vi "Pop-up password request.vi"(4 "error in (no error)":errorcluster, 7 "Filepath":path=path "C:/Projects - VSS/PART11 & DI TOOLKIT/passwords.log") -> (0 "error out":errorcluster, 1 "Activity log":T5 {"Epoch sec" format="%.2e"}, 2 "User access cluster":T3 {"Expire sec" format="%.2f"}, 3 "Valid password?":bool)   [LabVIEW 2013]
doc: "This is a pop-up panel which forces the user to enter a valid password or click cancel. It is a modal GUI.\n\nIt uses a filepath to an encrypted password file. If the user fails to enter a valid set of user ID and password within a set number of attempts (from the password file) the vi returns with valid password = F. \n\nIf there is a file read error then \"valid password?\" = F and a custom error code is returned (error not announced here). Conversely, incorrect user ID or password entries and expired passwords ARE announced in this vi.\n\nIt returns the User ID result, Security level (0 - 10), and an activty log of all failed and succesfull log-in attempts, which can be written to an activity log file by subsequent vis."
uses:
  User Access Type defs/Acitivity cluster array.ctl
  User Access Type defs/Acitivity cluster.ctl
  User Access Type defs/User access cluster.ctl
  User Access Type defs/Security level U8.ctl
  User Access Type defs/All users access configuration cluster.ctl
  User Access Type defs/User access cluster array.ctl
  <vilib>/Utility/miscctls.llb/LVPointTypeDef.ctl
panel:
  out "Access Configuration":T1 {"User array"."Expire sec" format="%.2f"}
  out "Lock user?":bool
  out "index":i32
  out "Password count":u8
  out "User ID count":u8
  out "State case":string
  in  "Password":string
  in  "Boolean 2":bool
  in  "Boolean":bool
  out "prompt":string="Enter a valid operator ID\nand password"
  in  "User ID":string
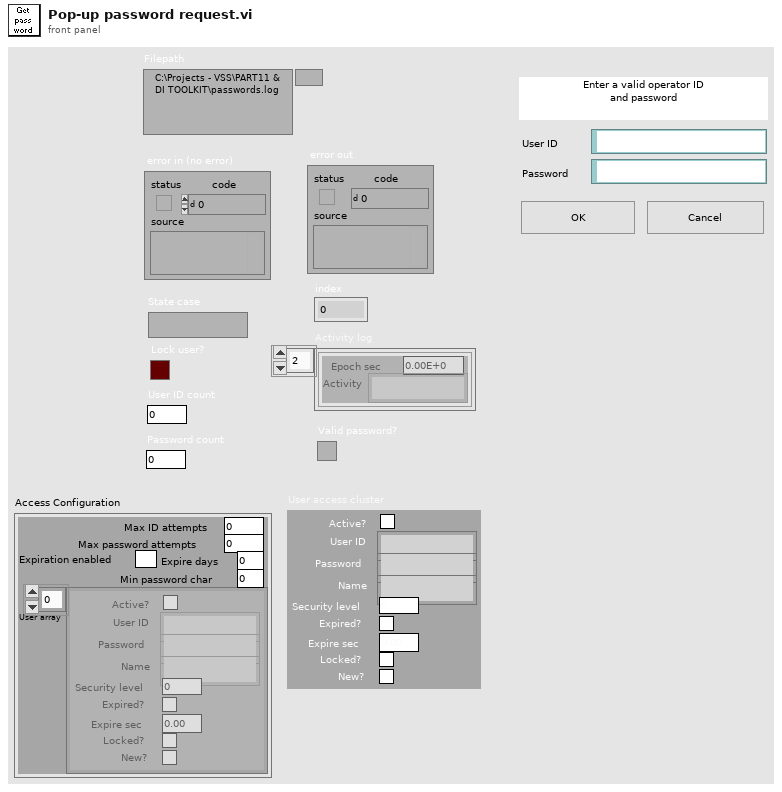
[diagram p1: front panel]
types:
  T1 = typedef "All users access configuration cluster.ctl" = cluster{"Max ID attempts":i32, "Max password attempts":i32, "Expiration enabled":bool, "Expire days":i32, "User array":T2, "Min password char":i32}
  T2 = typedef "User access cluster array.ctl" = T3[]
  T3 = typedef "User access cluster.ctl" = cluster{"Active?":bool, "User ID":string, "Password":string, "Name":string, "Security level":T4, "Expired?":bool, "Expire sec":dbl, "Locked?":bool, "New?":bool}
  T4 = typedef "Security level U8.ctl" = u8
  T5 = typedef "Acitivity cluster array.ctl" = T6[]
  T6 = typedef "Acitivity cluster.ctl" = cluster{"Epoch sec":dbl, "Activity":string}
  T7 = typedef "LVPointTypeDef.ctl" = cluster{"Horizontal":i16, "Vertical":i16}
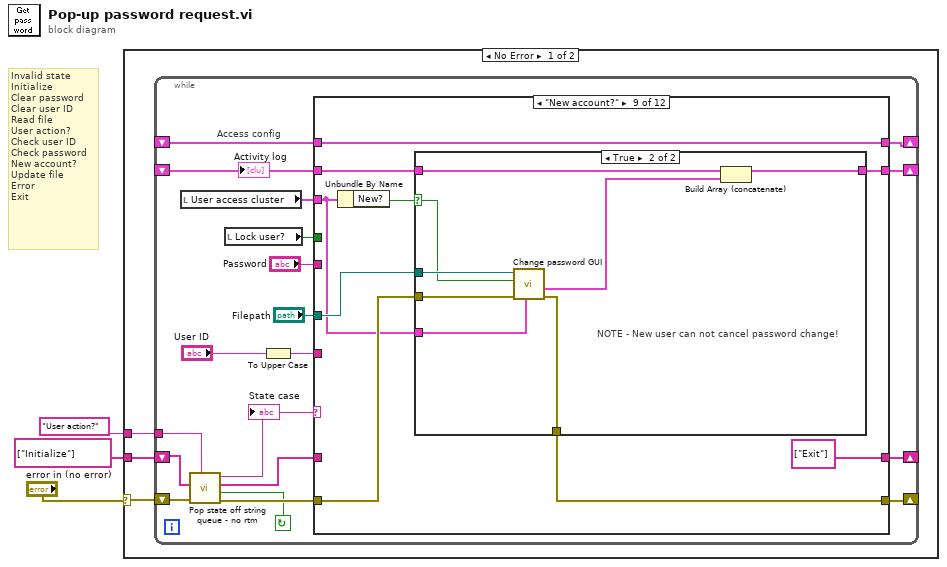
[diagram p0: block diagram]
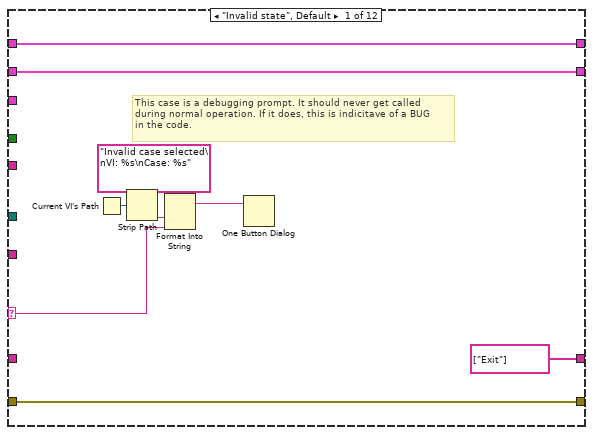
[diagram p2: hidden frame]
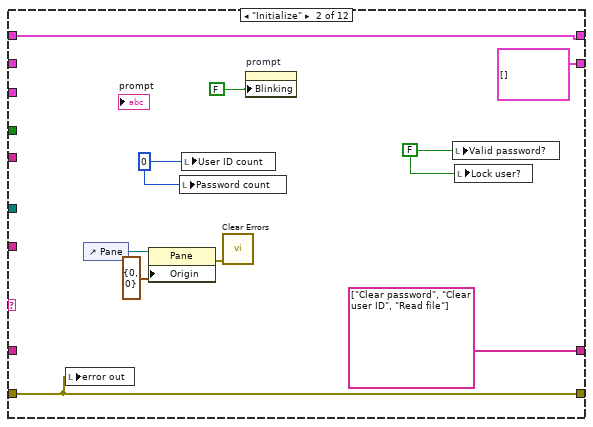
[diagram p3: hidden frame]
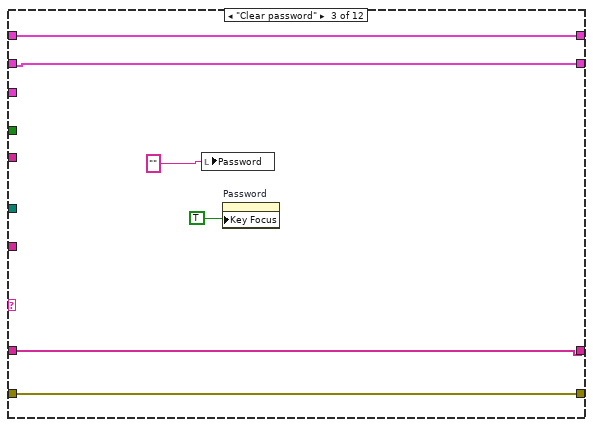
[diagram p4: hidden frame]
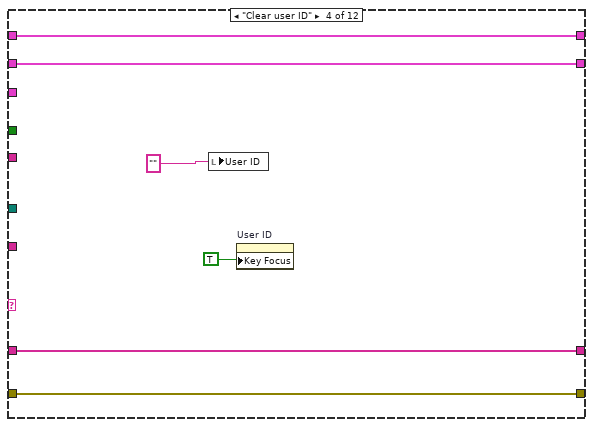
[diagram p5: hidden frame]
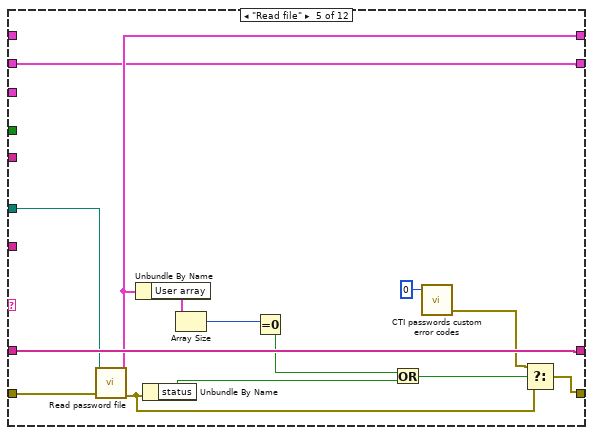
[diagram p6: hidden frame]
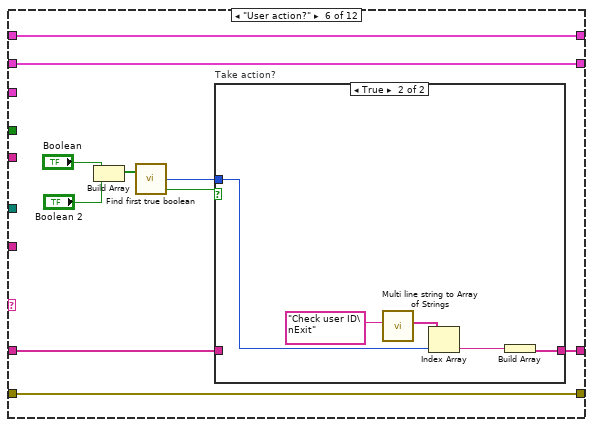
[diagram p7: hidden frame]
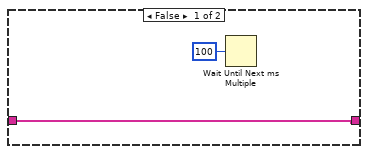
[diagram p8: hidden frame]
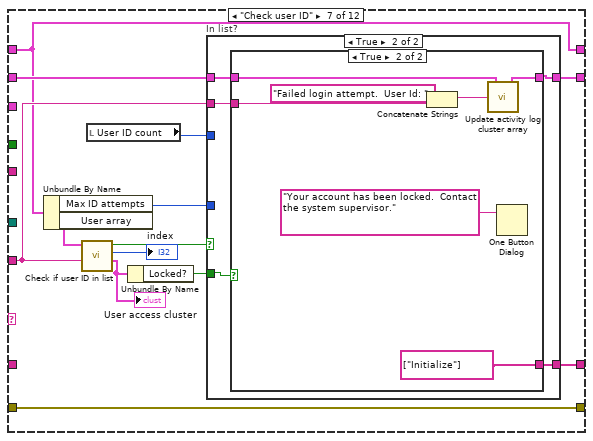
[diagram p9: hidden frame]
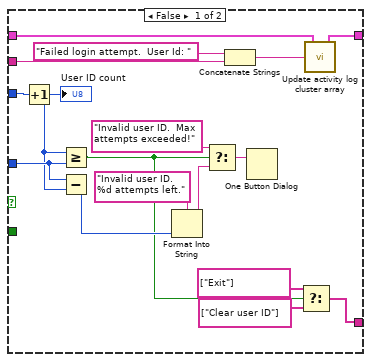
[diagram p10: hidden frame]
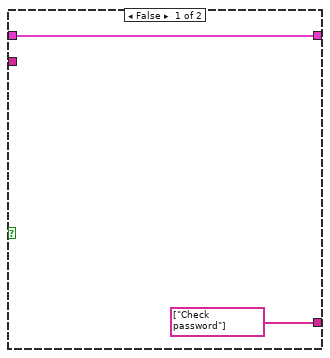
[diagram p11: hidden frame]
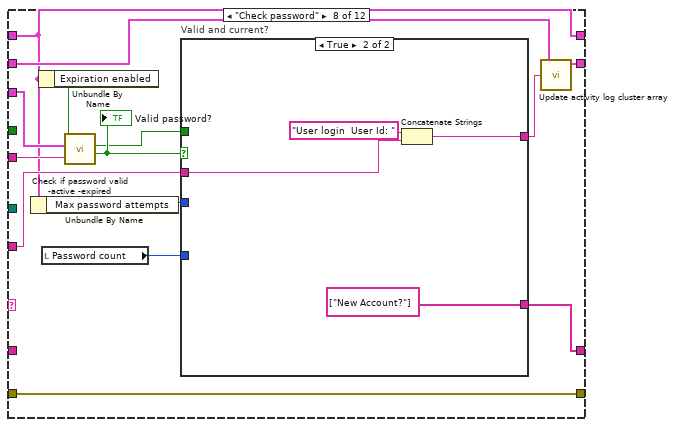
[diagram p12: hidden frame]
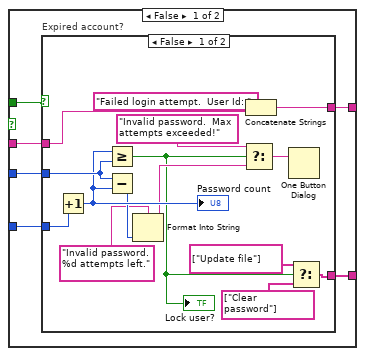
[diagram p13: hidden frame]
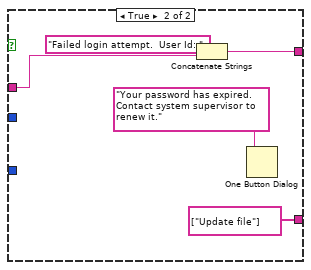
[diagram p14: hidden frame]
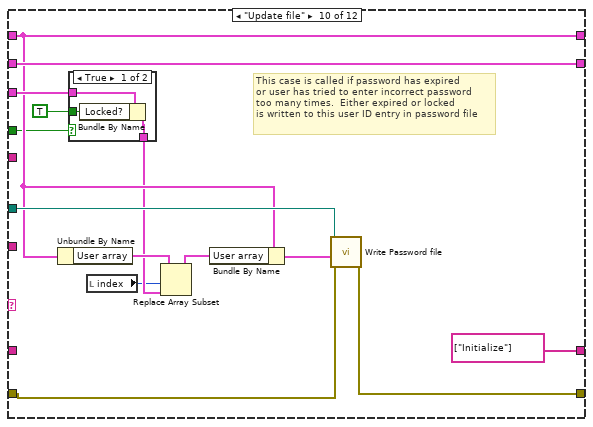
[diagram p16: hidden frame]
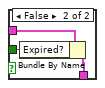
[diagram p17: hidden frame]
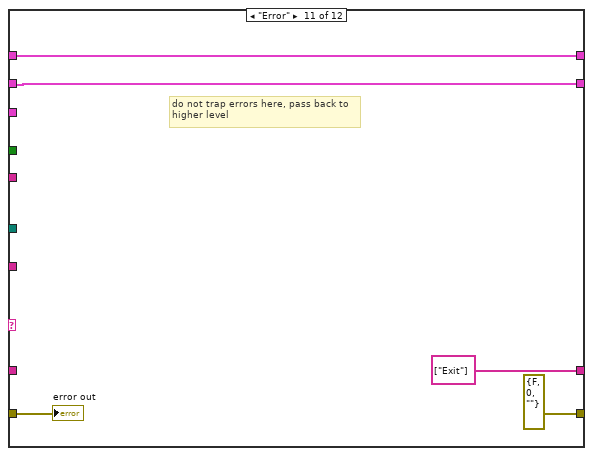
[diagram p18: hidden frame]
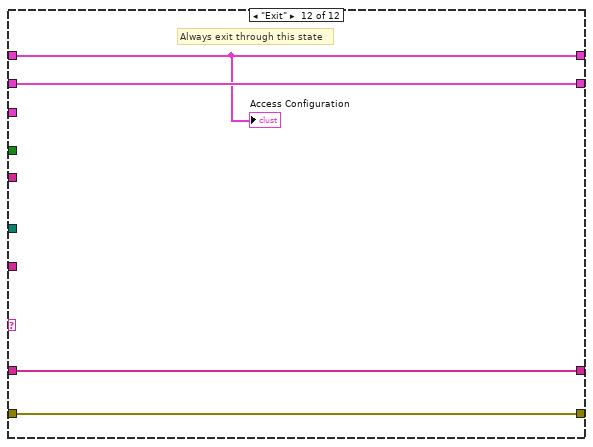
[diagram p19: hidden frame]
diagram:
  # "Invalid state\nInitialize\nClear password\nClear user ID\nRead file\nUser action?\nCheck user ID\nCheck password\nNew account?\nUpdate file\nError\nExit"
  n1 = case shown="No Error" "error in (no error)" {
    selector: "error in (no error)" -> [w6 _]
    tunnel: string[] ["Initialize"] ("State que out") -> [w5 _]
    tunnel: "User action?" ("Default state") -> [w4 _]
    frame No Error {
      n2 = while {
        tunnel: w4 -> [w17]
        shift-left: w5 -> [w21]
        shift-right: [w19] -> _
        shift-left: w6 -> [w25]
        shift-right: [w23] -> _
        shift-right: [w15] -> _
        shift-left: _ -> [w16]
        shift-right: [w14] -> _
        shift-left: _ -> [w13]
        stop <- w18 continue-if-true
        # "Access config"
        n3 = local read "User access cluster"() -> (w10:T3)
        n4 = call "Pop state off string queue - no rtm.vi"("Default state"=w17, "error in (no error)"=w25, "State que in"=w21) -> ("error out"=w24:errorcluster, "Not Exit?"=w18:bool, "State que out"=w20:string[], "State case"=w22:string)  [unwired: 5 out]
        "State case" <- w22
        n5 = local read "Lock user?"() -> (w8:bool)
        n6 = To Upper Case(1:"User ID") -> (0:w7:string)
        n7 = case shown="\"New account?\"" w22 {
          selector: w22 -> [w29 _ _ _ _ _ _ _ _ _ _ _]
          tunnel: [w34 w44 w50 w56 w63 w80 w100 w145 w178 w206 errorcluster {"status"=FALSE, "code"=0, "source"=""} ("error out") w222] -> w23
          tunnel: w24 -> [w34 w44 w50 w56 w69 w80 w100 w145 w179 w205 w217 w222]
          tunnel: [string[] ["Exit"] ("State que out") string[] ["Clear password", "Clear user ID", "Read file"] ("State que out") w46 w52 w70 w79 w97 w144 string[] ["Exit"] ("State que out") string[] ["Initialize"] ("State que out") string[] ["Exit"] ("State que out") w223] -> w19
          tunnel: w20 -> [_ _ w46 w52 w70 w71 _ _ _ _ _ w223]
          tunnel: [w27 w41 w48 w54 w67 w77 w91 w133 w184 w202 w215 w220] -> w15
          tunnel: w16 -> [w27 w41 w48 w54 _ w77 w91 w133 w184 w202 w215 w220]
          tunnel: w13 -> [w26 _ w47 w53 w57 w78 w94 w137 w181 w208 w216 w221]
          tunnel: [w26 T5 [] ("Activity log") w47 w53 w57 w78 w93 w136 w180 w208 w216 w221] -> w14
          tunnel: "Filepath" -> [_ _ _ _ w68 _ _ _ w177 w204 _ _]
          tunnel: w7 -> [_ _ _ _ _ _ w92 w141 _ _ _ _]
          tunnel: w10 -> [_ _ _ _ _ _ _ w139 w176 w203 _ _]
          tunnel: "Password" -> [_ _ _ _ _ _ _ w140 _ _ _ _]
          tunnel: w8 -> [_ _ _ _ _ _ _ _ _ w199 _ _]
          frame "Invalid state", Default {
            # "This case is a debugging prompt. It should never get called\nduring normal operation. If it does, this is indicitave of a BUG\nin the code."
            n8 = Current VI's Path() -> (path=w31:path)
            n9 = Strip Path(path=w31) -> (name=w30:string)  [unwired: 1 out]
            n10 = Format Into String(format string="Invalid case selected\nVI: %s\nCase: %s" ("message"), w30, w29) -> (resulting string=w32:string)  [unwired: 2 in, 1 out]
            n11 = One Button Dialog(message=w32) -> ()  [unwired: 2 out]
          }
          frame "Initialize" {
            w42 = u8 0 ("User ID count")
            w39 = FALSE ("Valid password?")
            n12 = local write "error out"(w44) -> ()
            n13 = control-ref of="Pane"() -> (w37:refnum<vi>)
            n14 = property class="Pane"(reference=w37, "Origin"=T7 {"Horizontal"=0, "Vertical"=0}) -> (error out=w35:errorcluster)  [unwired: 1 in, 1 out]
            n15 = local write "Password count"(w42) -> ()
            n16 = local write "User ID count"(w42) -> ()
            n17 = call <vilib>:"Clear Errors.vi"("error in (no error)"=w35) -> ()  [unwired: 7 out]
            n18 = property on="prompt" class="Str"("Blinking"=FALSE) -> ()  [unwired: 2 in, 2 out]
            n19 = local write "Valid password?"(w39) -> ()
            n20 = local write "Lock user?"(w39) -> ()
          }
          frame "Clear password" {
            n21 = local write "Password"("" ("Password")) -> ()
            n22 = property on="Password" class="Str"("Key Focus"=TRUE) -> ()  [unwired: 2 in, 2 out]
          }
          frame "Clear user ID" {
            n23 = local write "User ID"("" ("Password")) -> ()
            n24 = property on="User ID" class="Str"("Key Focus"=TRUE) -> ()  [unwired: 2 in, 2 out]
          }
          frame "Read file" {
            n25 = call "Read password file.vi"("error in (no error)"=w69, "file path"=w68) -> ("error out"=w64:errorcluster, "Access Configuration"=w67:T1)  [unwired: 8 out]
            n26 = Unbundle By Name(w67) -> ("User array"=w66:T2)
            n27 = Unbundle By Name(w64) -> ("status"=w61:bool)
            n28 = Array Size(array=w66) -> (size(s)=w65:i32)
            n29 = Equal To 0?(x=w65) -> (x = 0?=w62:bool)
            n30 = Or(x=w62, y=w61) -> (x .or. y?=w60:bool)
            n31 = call "CTI passwords custom error codes.vi"("error index"=0) -> ("error out"=w59:errorcluster)  [unwired: 1 in, 3 out]
            n32 = Select(t=w59, s=w60, f=w64) -> (s? t:f=w63:errorcluster)
          }
          frame "User action?" {
            n33 = Build Array("Boolean", "Boolean 2") -> (w74:bool[])
            n34 = call "Find first true boolean.vi"("Boolean Array IN"=w74) -> ("Index of first (T)"=w72:i32, "True found?"=w73:bool)  [unwired: 2 out]
            n35 = case "Take action?" shown="True" w73 {
              tunnel: [w82 w84] -> w79
              tunnel: w72 -> [_ w86]
              tunnel: w71 -> [w82 _]
              frame False {
                n36 = Wait Until Next ms Multiple(millisecond multiple=u32 100) -> ()  [unwired: 1 out]
              }
              frame True {
                n37 = call "Multi line string to Array of Strings.vi"("Multi Line String"="Check user ID\nExit") -> ("Array of Strings"=w87:string[])  [unwired: 6 out]
                n38 = Index Array(array=w87, index=w86) -> (element=w85:string)
                n39 = Build Array(w85) -> (w84:string[])
              }
            }
          }
          frame "Check user ID" {
            n40 = Unbundle By Name(w91) -> ("Max ID attempts"=w95:i32, "User array"=w99:T2)
            n41 = call "Check if user ID in list.vi"("User ID"=w92, "User array"=w99) -> ("User access cluster"=w90:T3, "index"=→"index":i32, "In list?"=w98:bool)  [unwired: 7 out]
            "User access cluster" <- w90
            n42 = local read "User ID count"() -> (w96:u8)
            n43 = Unbundle By Name(w90) -> ("Locked?"=w89:bool)
            n44 = case "In list?" shown="True" w98 {
              tunnel: [w108 w122] -> w97
              tunnel: w96 -> [w117 _]
              tunnel: w95 -> [w115 _]
              tunnel: [w106 w120] -> w93
              tunnel: w94 -> [w107 w121]
              tunnel: w92 -> [w103 w119]
              tunnel: w89 -> [_ w118]
              frame False {
                n45 = Increment(x=w117) -> (x+1=w114:u8)
                "User ID count" <- w114
                n46 = Greater Or Equal?(x=w114, y=w115) -> (x >= y?=w110:bool)
                n47 = Subtract(x=w115, y=w114) -> (x-y=w113:i32)
                n48 = Format Into String(format string="Invalid user ID.  %d attempts left." ("message"), w113) -> (resulting string=w111:string)  [unwired: 2 in, 1 out]
                n49 = Select(t="Invalid user ID.  Max attempts exceeded!" ("message"), s=w110, f=w111) -> (s? t:f=w105:string)
                n50 = Concatenate Strings("Failed login attempt.  User Id: ", w103) -> (w102:string)
                n51 = One Button Dialog(message=w105) -> ()  [unwired: 2 out]
                n52 = Select(t=string[] ["Exit"] ("State que out"), s=w110, f=string[] ["Clear user ID"] ("State que out")) -> (s? t:f=w108:string[])
                n53 = call "Update activity log cluster array.vi"("Activity description"=w102, "Activity log in"=w107) -> ("Activity log out"=w106:T5)  [unwired: 3 out]
              }
              frame True {
                n54 = case shown="True" w118 {
                  tunnel: [string[] ["Check password"] ("State que out") string[] ["Initialize"] ("State que out")] -> w122
                  tunnel: [w123 w129] -> w120
                  tunnel: w121 -> [w123 w130]
                  tunnel: w119 -> [_ w128]
                  frame False {
                  }
                  frame True {
                    n55 = Concatenate Strings("Failed login attempt.  User Id: ", w128) -> (w131:string)
                    n56 = call "Update activity log cluster array.vi"("Activity description"=w131, "Activity log in"=w130) -> ("Activity log out"=w129:T5)  [unwired: 3 out]
                    n57 = One Button Dialog(message="Your account has been locked.  Contact the system supervisor.") -> ()  [unwired: 2 out]
                  }
                }
              }
            }
          }
          frame "Check password" {
            n58 = Unbundle By Name(w133) -> ("Max password attempts"=w142:i32)
            n59 = Unbundle By Name(w133) -> ("Expiration enabled"=w132:bool)
            n60 = local read "Password count"() -> (w143:u8)
            n61 = call "Check if password valid -active -expired.vi"("Password"=w140, "User access cluster"=w139, "Expiration enabled?"=w132) -> ("Valid & current?"=w138:bool, "Expired?"=w134:bool)  [unwired: 1 in, 6 out]
            "Valid password?" <- w138
            n62 = case "Valid and current?" shown="True" w138 {
              tunnel: [w149 string[] ["New Account?"] ("State que out")] -> w144
              tunnel: w143 -> [w151 _]
              tunnel: w142 -> [w150 _]
              tunnel: w141 -> [w148 w173]
              tunnel: [w147 w172] -> w135
              tunnel: w134 -> [w146 _]
              frame False {
                n63 = case "Expired account?" shown="False" w146 {
                  tunnel: w151 -> [w166 _]
                  tunnel: w150 -> [w164 _]
                  tunnel: [w159 string[] ["Update file"] ("State que out")] -> w149
                  tunnel: w148 -> [w156 w170]
                  tunnel: [w154 w167] -> w147
                  frame False {
                    n64 = Increment(x=w166) -> (x+1=w163:u8)
                    "Password count" <- w163
                    n65 = Greater Or Equal?(x=w163, y=w164) -> (x >= y?=w153:bool)
                    "Lock user?" <- w153
                    n66 = Subtract(x=w164, y=w163) -> (x-y=w162:i32)
                    n67 = Format Into String(format string="Invalid password.  %d attempts left." ("message"), w162) -> (resulting string=w160:string)  [unwired: 2 in, 1 out]
                    n68 = Select(t="Invalid password.  Max attempts exceeded!" ("message"), s=w153, f=w160) -> (s? t:f=w158:string)
                    n69 = Concatenate Strings("Failed login attempt.  User Id: ", w156) -> (w154:string)
                    n70 = One Button Dialog(message=w158) -> ()  [unwired: 2 out]
                    n71 = Select(t=string[] ["Update file"] ("State que out"), s=w153, f=string[] ["Clear password"] ("State que out")) -> (s? t:f=w159:string[])
                  }
                  frame True {
                    n72 = Concatenate Strings("Failed login attempt.  User Id: ", w170) -> (w167:string)
                    n73 = One Button Dialog(message="Your password has expired.  Contact system supervisor to renew it.") -> ()  [unwired: 2 out]
                  }
                }
              }
              frame True {
                n74 = Concatenate Strings("User login  User Id: ", w173) -> (w172:string)
              }
            }
            n75 = call "Update activity log cluster array.vi"("Activity description"=w135, "Activity log in"=w137) -> ("Activity log out"=w136:T5)  [unwired: 3 out]
          }
          frame "New account?" {
            n76 = Unbundle By Name(w176) -> ("New?"=w182:bool)
            n77 = case shown="True" w182 {
              selector: w182 -> [_ w191]
              tunnel: [w186 w188] -> w180
              tunnel: w181 -> [w186 w189]
              tunnel: w179 -> [w185 w194]
              tunnel: [w185 w193] -> w178
              tunnel: w177 -> [_ w192]
              tunnel: w176 -> [_ w190]
              frame False {
              }
              frame True {
                # "NOTE - New user can not cancel password change!"
                n78 = call "Change password GUI.vi"("User access cluster in"=w190, "error in (no error)"=w194, "New user?"=w191, "Filepath"=w192) -> ("error out"=w193:errorcluster, "Activity log out"=w187:T5)  [unwired: 6 out]
                n79 = Build Array (concatenate)(w189, w187) -> (w188:T5)
              }
            }
          }
          frame "Update file" {
            # "This case is called if password has expired\nor user has tried to enter incorrect password\ntoo many times.  Either expired or locked\nis written to this user ID entry in password file"
            n80 = Unbundle By Name(w202) -> ("User array"=w201:T2)
            n81 = case shown="True" w199 {
              tunnel: w203 -> [w211 w214]
              tunnel: TRUE -> [w210 w213]
              tunnel: [w209 w212] -> w197
              frame True {
                n82 = Bundle By Name(cluster=w211, "Locked?"=w210) -> (w209:T3)
              }
              frame False {
                n83 = Bundle By Name(cluster=w214, "Expired?"=w213) -> (w212:T3)
              }
            }
            n84 = local read "index"() -> (w196:i32)
            n85 = Replace Array Subset(array=w201, new element=w197, index=w196) -> (w200:T2)
            n86 = Bundle By Name(cluster=w202, "User array"=w200) -> (w195:T1)
            n87 = call "Write Password file.vi"("error in (no error)"=w205, "Access Configuration"=w195, "Path"=w204) -> ("error out"=w206:errorcluster)  [unwired: 8 out]
          }
          frame "Error" {
            # "do not trap errors here, pass back to\nhigher level"
            "error out" <- w217
          }
          frame "Exit" {
            # "Always exit through this state"
            "Access Configuration" <- w220
          }
        }
        "Activity log" <- w13
      }
    }
    frame Error {
    }
  }
